vi "Read_Data_file.vi"(0 "Results file":path, 1 "Read Channel Names only":bool, 2 "Delete First Rows?":bool, 3 "Add Extra Channels?":bool, 5 "Template File":path, 7 "Run EnFlo Hub? (T)":bool=TRUE, 8 "Desired File Types":T1) -> (9 "Deleted Rows":string[][](array[string]), 10 "Row numbers":i32[](array[numeric]), 11 "Template File Out":path, 12 "Filetype":string, 14 "Results file Out":path, 15 "String Before":string, 16 "Ch names Out":string[](array[string]), 17 "Channel Values Out":string[][](array[string]), 18 "String After":string, 19 "Start Bytes":i32)   [LabVIEW 2022 SP3]
uses:
  Data_File_Type.ctl
  Globals/Meas_global.vi
panel:
  out "Case":string
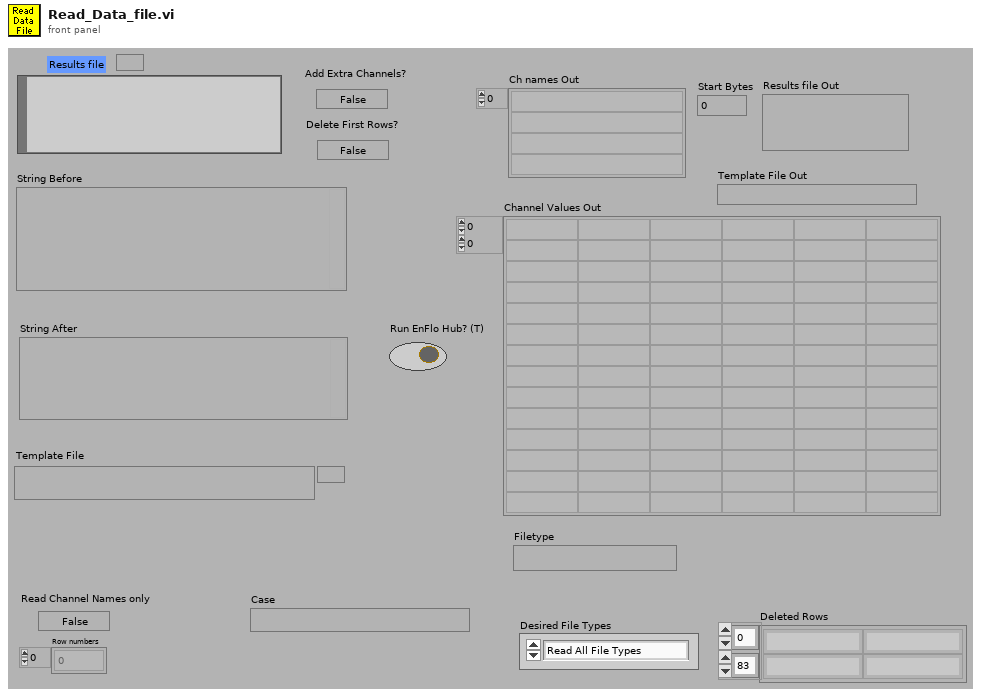
[diagram p1: front panel]
types:
  T1 = typedef "Data_File_Type.ctl" = enum16{"Read All File Types", "Results Files Only", "Raw Data Files Only", "Calibration Files Only", "Gas Desk Files Only", "Old Results Files Only", "Tabulated Data Files Only"}
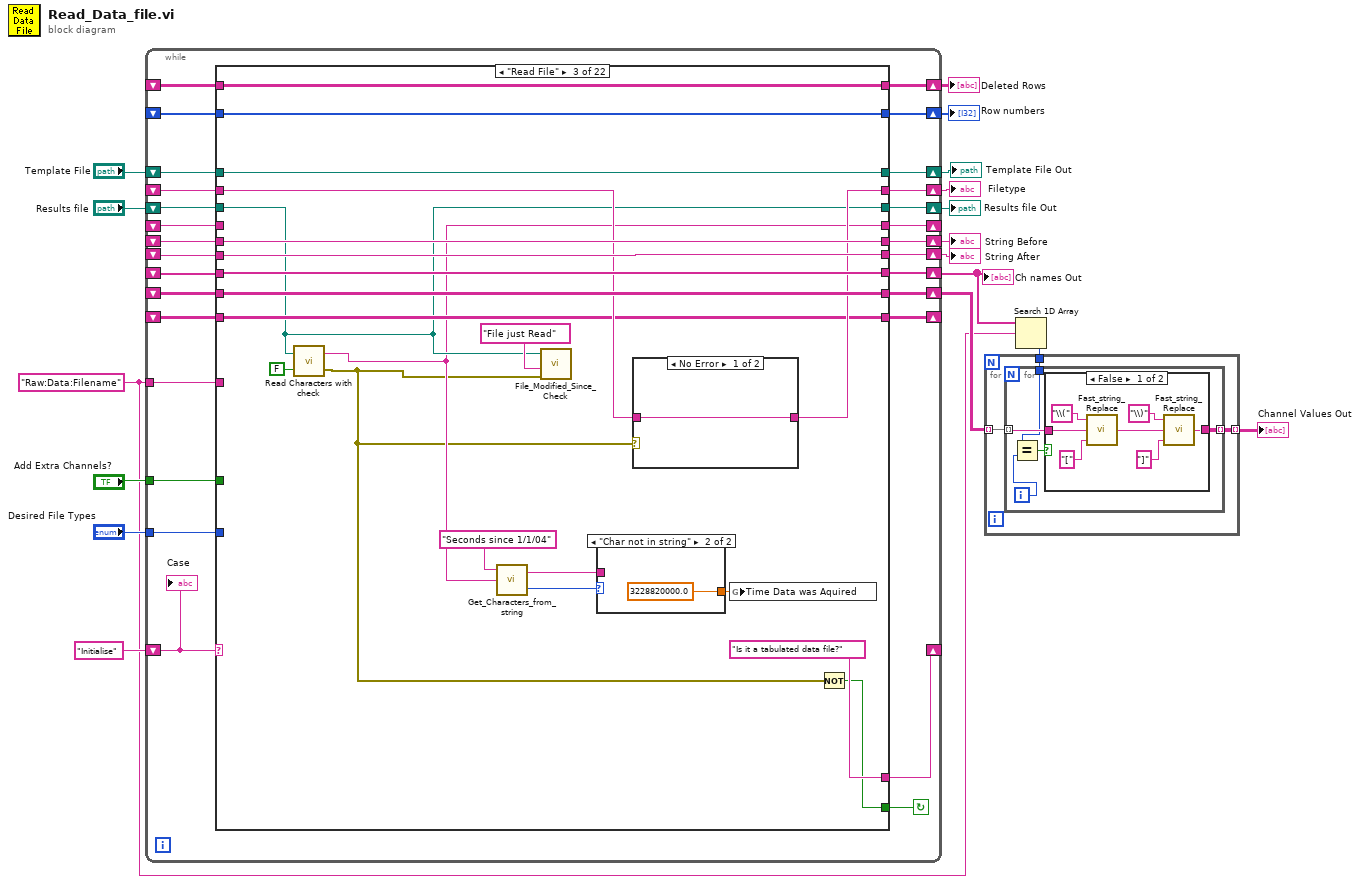
[diagram p0: block diagram]
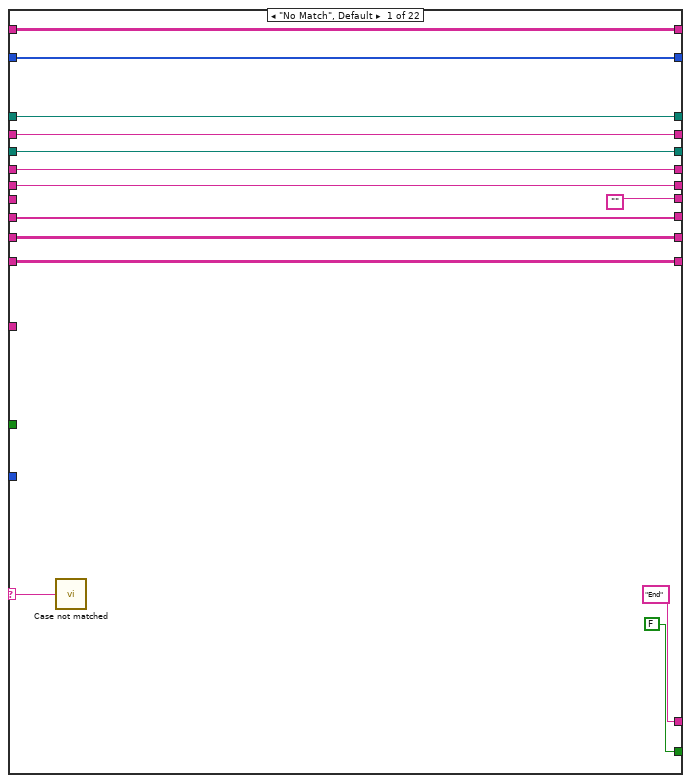
[diagram p3: hidden frame]
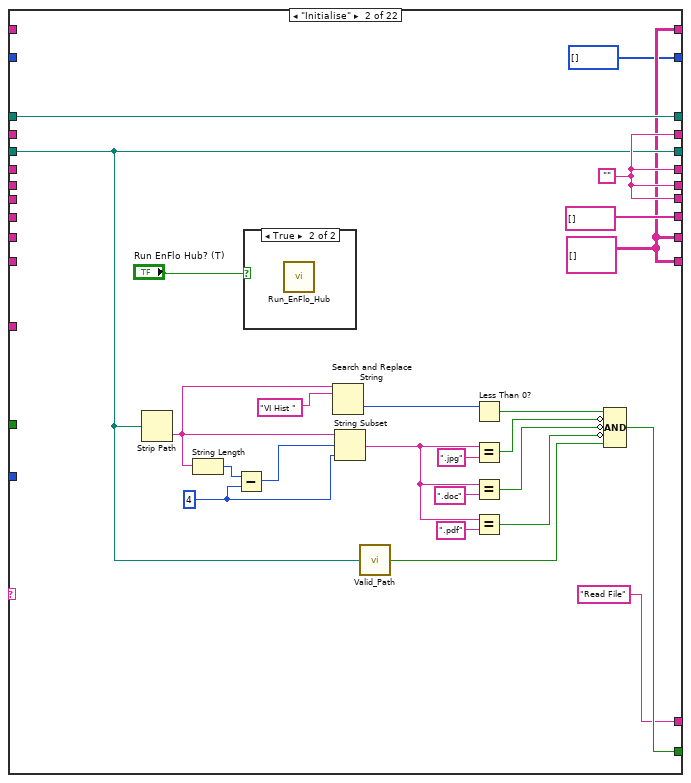
[diagram p4: hidden frame]
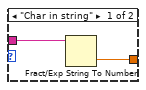
[diagram p6: hidden frame]
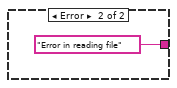
[diagram p7: hidden frame]
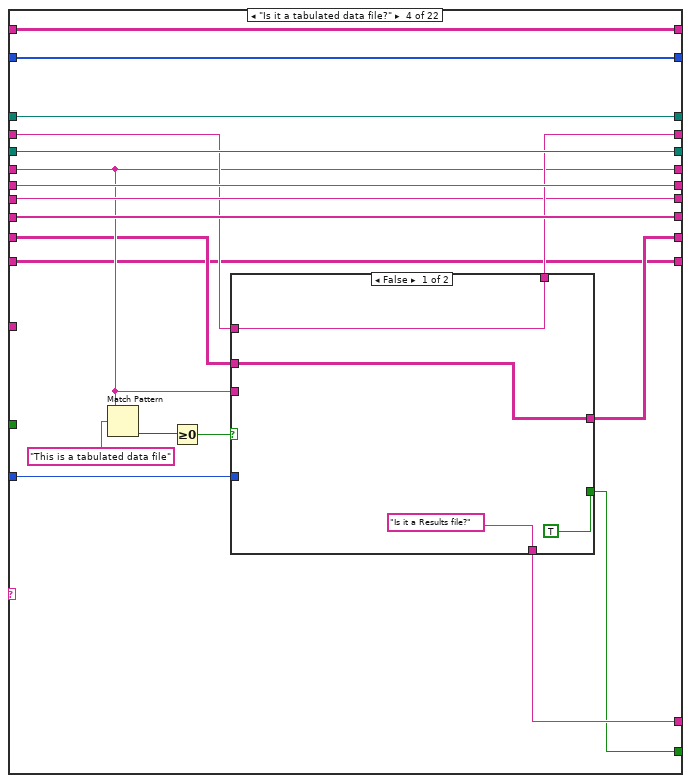
[diagram p8: hidden frame]
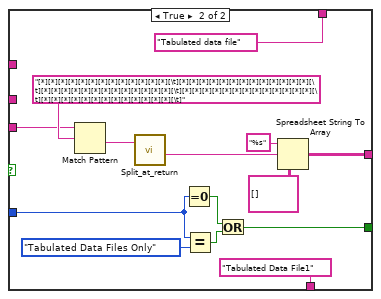
[diagram p9: hidden frame]
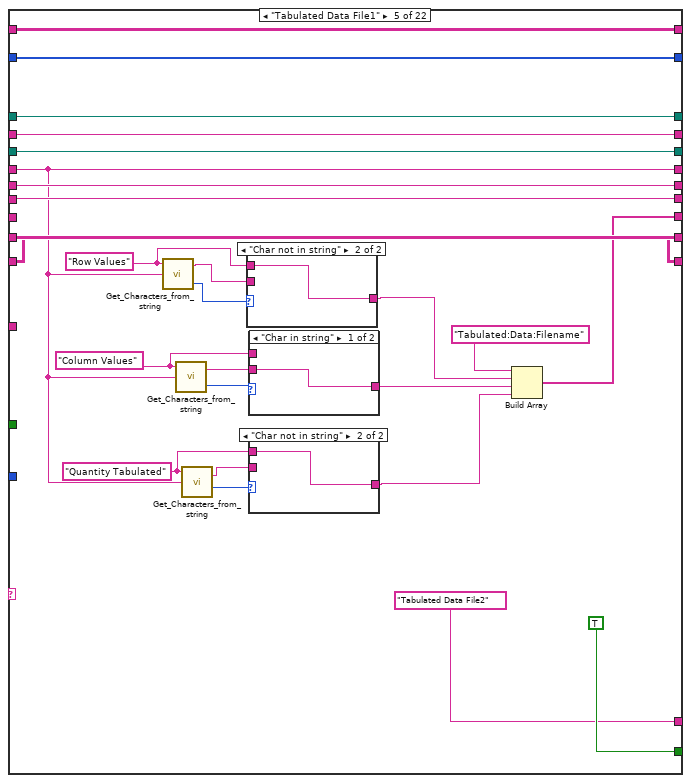
[diagram p10: hidden frame]
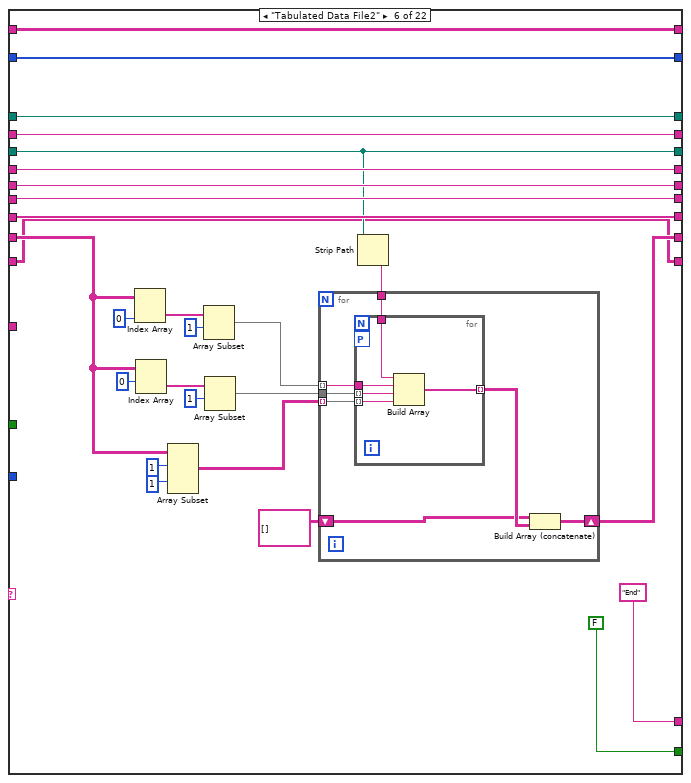
[diagram p14: hidden frame]
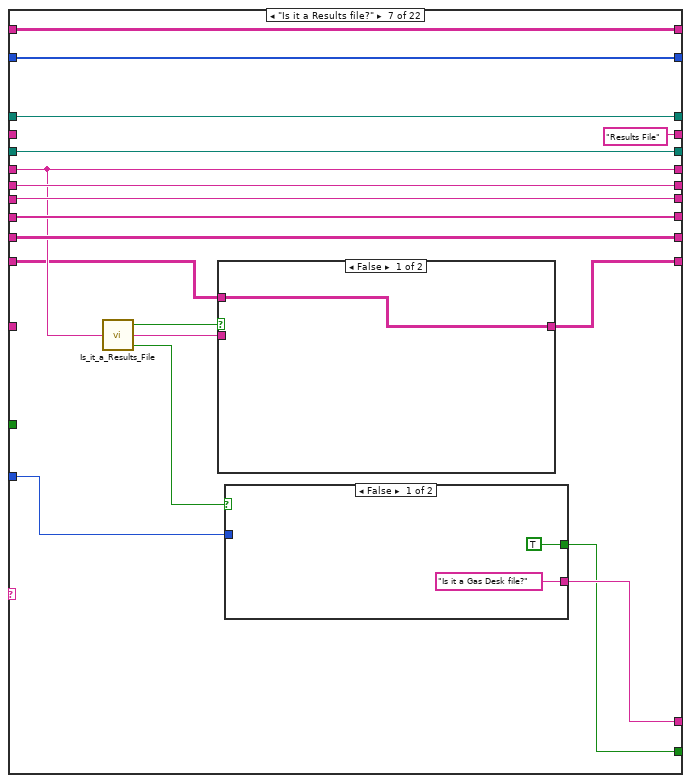
[diagram p15: hidden frame]
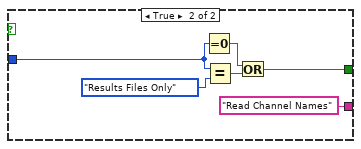
[diagram p16: hidden frame]
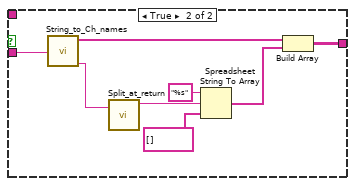
[diagram p17: hidden frame]
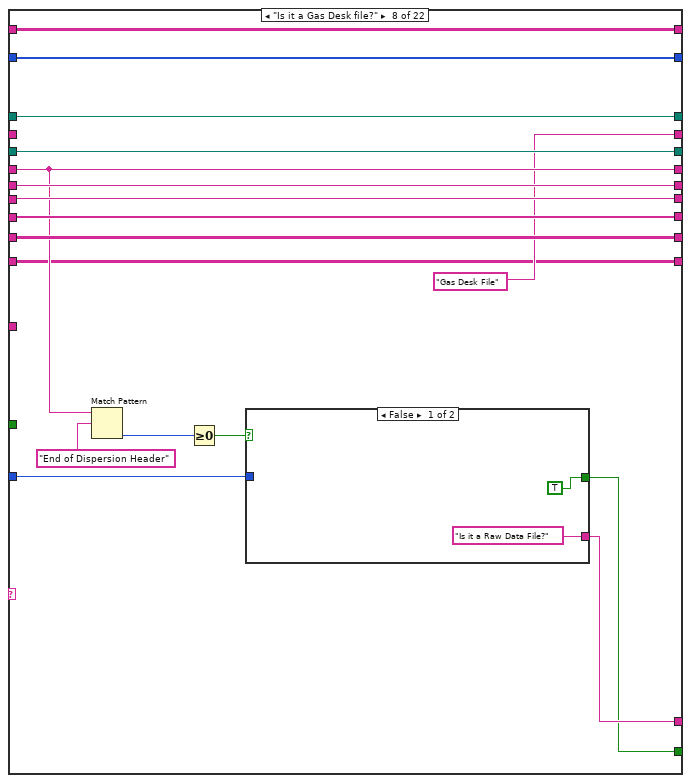
[diagram p18: hidden frame]
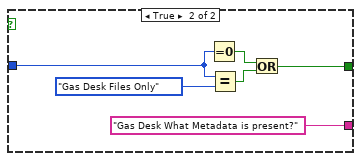
[diagram p19: hidden frame]
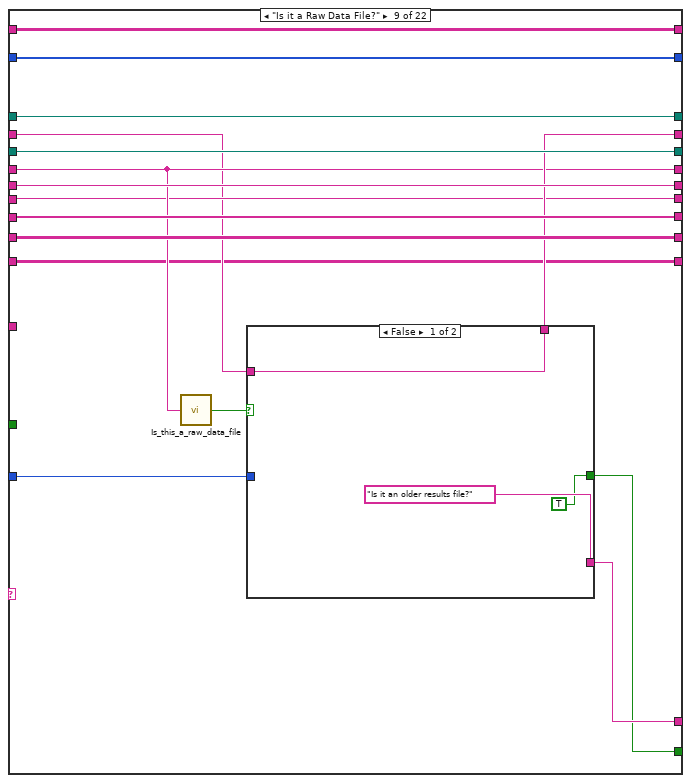
[diagram p20: hidden frame]
diagram:
  w2 = "Raw:Data:Filename"
  n1 = while {
    tunnel: "Add Extra Channels?" -> [w28]
    shift-left: _ -> [w32]
    shift-right: [w31] -> w16
    shift-left: "Results file" -> [w34]
    shift-right: [w33] -> w14
    shift-left: _ -> [w36]
    shift-right: [w35] -> w11
    shift-left: _ -> [w29]
    shift-right: [w37] -> w13
    shift-left: _ -> [w38]
    shift-right: [w39] -> _
    shift-left: "Initialise" -> [w42]
    shift-right: [w40] -> _
    shift-left: _ -> [w30]
    shift-right: [w44] -> w5
    shift-left: _ -> [w41]
    shift-right: [w45] -> w3
    shift-right: [w27] -> w10
    shift-left: "Template File" -> [w26]
    shift-right: [w24] -> w8
    shift-left: _ -> [w25]
    tunnel: "Desired File Types" -> [w23]
    shift-right: [w22] -> w6
    shift-left: _ -> [w21]
    shift-right: [w20] -> _
    shift-left: _ -> [w19]
    tunnel: w2 -> [w18]
    stop <- w43 continue-if-true
    n2 = case shown="\"Read File\"" w42 {
      selector: w42 -> [w47 _ _ _ _ _ _ _ _ _ _ _ _ _ _ _ _ _ _ _ _ _]
      tunnel: [w58 string[] [] ("Extra Channel Names") w103 w128 w154 w205 w235 w269 w293 w321 w355 w389 w410 w449 w477 w479 w560 w604 w654 w679 w702 w728] -> w45
      tunnel: [w57 w61 w102 w117 w172 w194 w234 w268 w292 w320 w354 w388 w409 w448 w476 w499 w566 w621 w653 w674 w696 w725] -> w44
      tunnel: [FALSE ("Results File?") w73 w99 w112 TRUE ("Results File?") FALSE ("Results File?") w226 w255 w281 w307 w341 w381 TRUE ("Results File?") TRUE ("Results File?") TRUE ("Results File?") w487 TRUE ("Results File?") TRUE ("Results File?") FALSE ("Results File?") TRUE ("Results File?") w697 FALSE ("Results File?")] -> w43
      tunnel: w41 -> [w58 _ w103 w128 _ w205 w235 w269 w293 w321 w355 w389 w410 w449 w477 _ w560 w605 w658 w679 w702 w730]
      tunnel: ["End" "Read File" "Is it a tabulated data file?" w124 "Tabulated Data File2" ("f") "End" ("f") w233 w256 w288 w316 "Read Channel Names" ("f") "Read Channel Names" ("f") w395 "Read Channel Names" ("f") "Read Channel Names" ("f") w490 "Does template file exist?" ("f") w616 "End" ("f") "Delete First Row?" ("f") "Add Extra Channels of data" ("f") "End" ("f")] -> w40
      tunnel: [w55 w82 w86 w118 w165 w201 w228 w262 w286 w311 w350 w377 w397 w428 w460 w492 w561 w620 w659 w672 w704 w732] -> w39
      tunnel: w38 -> [w55 _ _ w118 w165 w201 w228 w262 w286 w311 w350 w384 w396 w428 w460 w494 w561 w620 w659 w672 w704 w732]
      tunnel: [w54 w82 w101 w126 w170 w204 w229 w265 w290 w318 w353 w386 w406 w445 w474 w493 w558 w619 w662 w678 w707 w736] -> w37
      tunnel: w36 -> [_ _ w100 w123 w168 w202 w231 w266 w285 w315 w352 _ w407 w446 w475 w498 w565 w618 w661 w677 w706 w735]
      tunnel: ["" w82 w100 w123 w168 w202 w231 w266 w285 w315 w352 w374 w407 w446 w475 w498 w565 w618 w661 w677 w706 w735] -> w35
      tunnel: w34 -> [w53 w71 w87 w127 w171 w184 w232 w267 w291 w319 w335 w387 w408 w447 w456 w497 w564 w602 w657 w671 w703 w731]
      tunnel: [w53 w71 w87 w127 w171 w184 w232 w267 w291 w319 w335 w387 w408 w447 w456 w497 w564 w602 w657 w671 w703 w731] -> w33
      tunnel: w32 -> [w51 _ w97 w122 w167 w200 _ _ w284 w314 _ w380 w394 w443 w472 w496 w563 w617 w656 w668 w701 w734]
      tunnel: [w51 w82 w98 w125 w167 w200 "Results File" "Gas Desk File" w289 w317 w340 w380 w394 w443 w472 w496 w563 w617 w656 w668 w701 w734] -> w31
      tunnel: w30 -> [w57 _ w102 w116 w172 w193 w234 w268 w292 w320 w354 w388 w409 w448 w476 w499 w566 w621 _ _ w700 w727]
      tunnel: w29 -> [w54 _ w101 w126 w170 w204 w229 w265 w290 w318 w353 w386 w406 w445 w474 _ w558 w619 w662 w678 w707 w736]
      tunnel: w28 -> [_ _ _ _ _ _ _ _ _ _ w342 _ _ _ _ _ _ _ _ _ w692 _]
      tunnel: [w50 w72 w96 w115 w150 w182 w224 w260 w283 w309 w339 w371 w393 w426 w455 w488 w557 w599 w652 w667 w683 w724] -> w27
      tunnel: w26 -> [w50 w72 w96 w115 w150 w182 w224 w260 w283 w309 w339 w371 w393 w426 w455 w488 w557 w599 w651 w667 w683 w724]
      tunnel: [w49 i32[] [] ("Row numbers") w95 w114 w149 w181 w223 w259 w282 w308 w338 w370 w392 w425 w454 w483 w556 w612 w650 w666 w684 w723] -> w24
      tunnel: w25 -> [w49 _ w95 w114 w149 w181 w223 w259 w282 w308 w338 w370 w392 w425 w454 w483 w556 w612 _ w666 _ w723]
      tunnel: w23 -> [_ _ _ w113 _ _ w221 w258 w280 w306 w337 _ _ _ _ _ _ _ _ _ _ _]
      tunnel: [w48 w61 w90 w111 w148 w180 w220 w254 w279 w305 w333 w369 w391 w424 w453 w482 w555 w603 w649 w665 w691 w722] -> w22
      tunnel: w21 -> [w48 _ w90 w111 w148 w180 w220 w254 w279 w305 w333 w369 w391 w424 w453 w482 w555 w603 _ w665 w690 w722]
      tunnel: [w46 w61 w89 w110 w147 w179 w219 w253 w278 w304 w332 w368 w390 w421 w450 w481 w553 w595 w648 w664 w688 w718] -> w20
      tunnel: w19 -> [w46 _ w89 w110 w147 w179 w218 w253 w278 w304 w332 w368 w390 _ _ w481 w554 w591 w648 w664 w688 w718]
      tunnel: w18 -> [_ _ _ _ _ _ _ _ _ _ _ _ _ _ _ _ w552 _ _ _ _ _]
      frame "No Match", Default {
        n3 = call "Case not matched.vi"("Case Name not Matched"=w47) -> ()
      }
      frame "Initialise" {
        w80 = 4 ("length (rest)")
        w82 = ""
        w61 = string[][] [] ("Channel Values")
        n4 = Strip Path(path=w71) -> (name=w78:string)  [unwired: 1 out]
        n5 = String Length(string=w78) -> (length=w81:i32)
        n6 = Subtract(x=w81, y=w80) -> (x-y=w79:i32)
        n7 = case shown="True" "Run EnFlo Hub? (T)" {
          frame False {
          }
          frame True {
            n8 = call "Run_EnFlo_Hub.vi"() -> ()  [unwired: 1 in, 7 out]
          }
        }
        n9 = Search and Replace String(input string=w78, search string="VI Hist ") -> (offset past replacement=w76:i32)  [unwired: 1 in, 8 out]
        n10 = String Subset(string=w78, offset (0)=w79, length (rest)=w80) -> (substring=w66:string)
        n11 = call "Valid_Path.vi"("Filename"=w71) -> ("Valid Path?"=w63:bool)
        n12 = Less Than 0?(x=w76) -> (x < 0?=w74:bool)
        n13 = Equal?(x=w66, y=".jpg") -> (x = y?=w75:bool)
        n14 = Equal?(x=w66, y=".doc") -> (x = y?=w69:bool)
        n15 = Equal?(x=w66, y=".pdf") -> (x = y?=w65:bool)
        n16 = Compound Arithmetic op=AND(w74, invert w75, invert w69, invert w65, w63) -> (w73:bool)
      }
      frame "Read File" {
        n17 = call "Read Characters with check.vi"("Call EnFlo Error Handler?"=FALSE, "file (use dialog)"=w87) -> ("error out"=w85:errorcluster, "Read String"=w86:string)
        n18 = call "Get_Characters_from_string.vi"("Input string"=w86, "Variable name"="Seconds since 1/1/04") -> ("Status"=w91:enum16{"Char in string", "Char not in string"}, "Value"=w93:string)  [unwired: 1 in]
        n19 = call "File_Modified_Since_Check.vi"("error in"=w85, "mode"="File just Read", "File Path"=w87) -> ()  [unwired: 5 in, 2 out]
        n20 = case shown="\"Char not in string\"" w91 {
          tunnel: w93 -> [w106 _]
          tunnel: [w105 3228820000.0 ("y")] -> w92
          frame "Char in string" {
            n21 = Fract/Exp String To Number(string=w106) -> (number=w105:dbl)  [unwired: 4 out]
          }
          frame "Char not in string" {
          }
        }
        n22 = case shown="No Error" w85 {
          tunnel: [w108 "Error in reading file"] -> w98
          tunnel: w97 -> [w108 _]
          frame No Error {
          }
          frame Error {
          }
        }
        n23 = global write "Meas_global.vi" "Time Data was Aquired"(w92) -> ()
        n24 = Not(x=w85) -> (.not. x?=w99:bool)
      }
      frame "Is it a tabulated data file?" {
        n25 = Match Pattern(string=w118, regular expression="This is a tabulated data file") -> (offset past match=w121:i32)  [unwired: 4 out]
        n26 = Greater Or Equal To 0?(x=w121) -> (x >= 0?=w120:bool)
        n27 = case shown="False" w120 {
          tunnel: [w132 "Tabulated data file"] -> w125
          tunnel: ["Is it a Results file?" "Tabulated Data File1" ("f")] -> w124
          tunnel: w122 -> [w132 _]
          tunnel: w118 -> [_ w143]
          tunnel: [w131 w140] -> w117
          tunnel: w116 -> [w131 _]
          tunnel: w113 -> [_ w136]
          tunnel: [TRUE ("Results File?") w133] -> w112
          frame False {
          }
          frame True {
            n28 = Match Pattern(string=w143, regular expression="[*][*][*][*][*][*][*][*][*][*][*][*][*][\t][*][*][*][*][*][*][*][*][*][*][*][*][*][\t][*][*][*][*][*][*][*][*][*][*][*][*][*][\t][*][*][*][*][*][*][*][*][*][*][*][*][*][\t][*][*][*][*][*][*][*][*][*][*][*][*][*][\t]" ("String")) -> (after substring=w139:string)  [unwired: 4 out]
            n29 = call "Split_at_return.vi"("String"=w139) -> ("after substring"=w138:string)  [unwired: 1 in, 3 out]
            n30 = Equal To 0?(x=w136) -> (x = 0?=w134:bool)
            n31 = Equal?(x=w136, y=Data_File_Type."Tabulated Data Files Only" ("Desired File Types")) -> (x = y?=w135:bool)
            n32 = Or(x=w134, y=w135) -> (x .or. y?=w133:bool)
            n33 = Spreadsheet String To Array(format string="%s", spreadsheet string=w138, array type (2D Dbl)=string[][] [] ("Channel Values")) -> (array=w140:string[][])  [unwired: 1 out]
          }
        }
      }
      frame "Tabulated Data File1" {
        w153 = "Row Values" ("Variable name")
        w152 = "Column Values" ("Variable name")
        w159 = "Quantity Tabulated" ("Variable name")
        n34 = call "Get_Characters_from_string.vi"("Input string"=w165, "Variable name"=w153) -> ("Status"=w157:enum16{"Char in string", "Char not in string"}, "Value"=w158:string)  [unwired: 1 in]
        n35 = call "Get_Characters_from_string.vi"("Input string"=w165, "Variable name"=w152) -> ("Status"=w164:enum16{"Char in string", "Char not in string"}, "Value"=w163:string)  [unwired: 1 in]
        n36 = call "Get_Characters_from_string.vi"("Input string"=w165, "Variable name"=w159) -> ("Status"=w161:enum16{"Char in string", "Char not in string"}, "Value"=w160:string)  [unwired: 1 in]
        n37 = case shown="\"Char not in string\"" w157 {
          tunnel: w158 -> [w175 _]
          tunnel: [w175 w176] -> w156
          tunnel: w153 -> [_ w176]
          frame "Char in string" {
          }
          frame "Char not in string" {
          }
        }
        n38 = case shown="\"Char in string\"" w164 {
          tunnel: w163 -> [w177 _]
          tunnel: [w177 w178] -> w162
          tunnel: w152 -> [_ w178]
          frame "Char in string" {
          }
          frame "Char not in string" {
          }
        }
        n39 = case shown="\"Char not in string\"" w161 {
          tunnel: w160 -> [w173 _]
          tunnel: [w173 w174] -> w155
          tunnel: w159 -> [_ w174]
          frame "Char in string" {
          }
          frame "Char not in string" {
          }
        }
        n40 = Build Array("Tabulated:Data:Filename", w156, w162, w155) -> (w154:string[])
      }
      frame "Tabulated Data File2" {
        n41 = Index Array(array=w193, index (col)=0 ("index (row)")) -> (element=w188:string[])  [unwired: 1 in]
        n42 = Index Array(array=w193, index (row)=0) -> (element=w192:string[])  [unwired: 1 in]
        n43 = Array Subset(array=w193, index (row)=1 ("index"), index (col)=1 ("index")) -> (w196:string[][])  [unwired: 2 in]
        n44 = Array Subset(array=w188, index=1) -> (w187:string[])  [unwired: 1 in]
        n45 = Array Subset(array=w192, index=1) -> (w189:string[])  [unwired: 1 in]
        n46 = Strip Path(path=w184) -> (name=w183:string)  [unwired: 1 out]
        n47 = for {
          tunnel: w187 -> [w212] mode=indexing
          tunnel: w189 -> [w211]
          tunnel: w196 -> [w210] mode=indexing
          shift-right: [w207] -> w194
          shift-left: string[][] [] -> [w208]
          tunnel: w183 -> [w206]
          n48 = for {
            tunnel: w212 -> [w217]
            tunnel: w211 -> [w216] mode=indexing
            tunnel: w210 -> [w215] mode=indexing
            tunnel: [w214] -> w209 mode=indexing
            tunnel: w206 -> [w213]
            workers-P: _ -> [_]
            n49 = Build Array(w213, w217, w216, w215) -> (w214:string[])
          }
          n50 = Build Array (concatenate)(w208, w209) -> (w207:string[][])
        }
      }
      frame "Is it a Results file?" {
        n51 = call "Is_it_a_Results_File.vi"("character string"=w228) -> ("Contain DB Header Info"=w227:bool, "Header String"=w222:string, "Results File?"=w225:bool)
        n52 = case shown="False" w227 {
          tunnel: w222 -> [_ w248]
          tunnel: [w244 w245] -> w219
          tunnel: w218 -> [w244 _]
          frame False {
          }
          frame True {
            n53 = call "String_to_Ch_names.vi"("Spreadsheet string"=w248) -> ("Ch names"=w247:string[], "String After names"=w251:string)  [unwired: 2 out]
            n54 = call "Split_at_return.vi"("String"=w251) -> ("before substring"=w252:string)  [unwired: 1 in, 3 out]
            n55 = Spreadsheet String To Array(format string="%s", spreadsheet string=w252, array type (2D Dbl)=string[] [] ("Channel Values")) -> (array=w246:string[])  [unwired: 1 out]
            n56 = Build Array(w247, w246) -> (w245:string[][])
          }
        }
        n57 = case shown="False" w225 {
          tunnel: ["Is it a Gas Desk file?" "Read Channel Names"] -> w233
          tunnel: w221 -> [_ w240]
          tunnel: [TRUE w238] -> w226
          frame False {
          }
          frame True {
            n58 = Equal To 0?(x=w240) -> (x = 0?=w241:bool)
            n59 = Equal?(x=w240, y=Data_File_Type."Results Files Only" ("Desired File Types")) -> (x = y?=w242:bool)
            n60 = Or(x=w241, y=w242) -> (x .or. y?=w238:bool)
          }
        }
      }
      frame "Is it a Gas Desk file?" {
        n61 = Match Pattern(string=w262, regular expression="End of Dispersion Header") -> (offset past match=w264:i32)  [unwired: 4 out]
        n62 = Greater Or Equal To 0?(x=w264) -> (x >= 0?=w257:bool)
        n63 = case shown="False" w257 {
          tunnel: ["Is it a Raw Data File?" "Gas Desk What Metadata is present?"] -> w256
          tunnel: w258 -> [_ w274]
          tunnel: [TRUE w272] -> w255
          frame False {
          }
          frame True {
            n64 = Equal To 0?(x=w274) -> (x = 0?=w275:bool)
            n65 = Equal?(x=w274, y=Data_File_Type."Gas Desk Files Only" ("Desired File Types")) -> (x = y?=w276:bool)
            n66 = Or(x=w275, y=w276) -> (x .or. y?=w272:bool)
          }
        }
      }
      frame "Is it a Raw Data File?" {
        n67 = call "Is_this_a_raw_data_file.vi"("character string"=w286) -> ("Raw Dat File?"=w287:bool)  [unwired: 2 out]
        n68 = case shown="False" w287 {
          tunnel: [w295 "Raw Data File"] -> w289
          tunnel: ["Is it an older results file?" ("f") "Does Raw data file Contain ADAM data?" ("f")] -> w288
          tunnel: w284 -> [w295 _]
          tunnel: [TRUE ("Results File?") w298] -> w281
          tunnel: w280 -> [_ w299]
          frame False {
          }
          frame True {
            n69 = Equal To 0?(x=w299) -> (x = 0?=w301:bool)
            n70 = Equal?(x=w299, y=Data_File_Type."Raw Data Files Only" ("Desired File Types")) -> (x = y?=w300:bool)
            n71 = Or(x=w301, y=w300) -> (x .or. y?=w298:bool)
          }
        }
      }
      frame "Is it an older results file?" {
        n72 = Match Pattern(string=w311, regular expression="Date of meas\tTime of meas") -> (offset past match=w312:i32)  [unwired: 4 out]
        n73 = Greater Or Equal To 0?(x=w312) -> (x >= 0?=w310:bool)
        n74 = case shown="False" w310 {
          tunnel: [w324 "Older Results File"] -> w317
          tunnel: ["Is it a calibration file?" ("f") "Read Channel Names" ("f")] -> w316
          tunnel: w314 -> [w324 _]
          tunnel: [TRUE ("Results File?") w326] -> w307
          tunnel: w306 -> [_ w325]
          frame False {
          }
          frame True {
            n75 = Equal To 0?(x=w325) -> (x = 0?=w329:bool)
            n76 = Equal?(x=w325, y=Data_File_Type."Old Results Files Only" ("Desired File Types")) -> (x = y?=w328:bool)
            n77 = Or(x=w329, y=w328) -> (x .or. y?=w326:bool)
          }
        }
      }
      frame "Is it a calibration file?" {
        w349 = FALSE  # Show Dialog?
        n78 = Format Into String(format string="Data File   %s", w335) -> (resulting string=w334:string)  [unwired: 2 in, 1 out]
        n79 = call "2D_array_from_string.vi"("String Name"=w334, "Show Dialog?"=w349, "Input string"=w350, "Array title"="Calib points label") -> ("2D data array"=w348:dbl[][])
        n80 = Array Size(array=w348) -> (size(s)=w347:i32[])
        n81 = Index Array(array=w347, index=0 ("Index")) -> (element=w345:i32)
        n82 = Greater Than 0?(x=w345) -> (x > 0?=w343:bool)
        n83 = case shown="False" w343 {
          tunnel: w342 -> [_ w367]
          tunnel: [w356 w359] -> w341
          tunnel: ["File with no header" "Calibration File"] -> w340
          tunnel: w337 -> [w357 w363]
          frame False {
            n84 = Equal To 0?(x=w357) -> (x = 0?=w356:bool)
          }
          frame True {
            n85 = Not(x=w367) -> (.not. x?=w360:bool)
            n86 = Equal To 0?(x=w363) -> (x = 0?=w365:bool)
            n87 = Equal?(x=w363, y=Data_File_Type."Calibration Files Only" ("Desired File Types")) -> (x = y?=w364:bool)
            n88 = Or(x=w365, y=w364) -> (x .or. y?=w361:bool)
            n89 = Or(x=w360, y=w361) -> (x .or. y?=w359:bool)
          }
        }
      }
      frame "Does Raw data file Contain ADAM data?" {
        w372 = "\r\n"
        w375 = "Raw data header Start"
        n90 = Match Pattern(string=w384, regular expression=w375) -> (before substring=w378:string, after substring=w373:string)  [unwired: 3 out]
        n91 = Match Pattern(string=w378, regular expression="[*][*][*][*][*][*][*][*][*][*][*][*][*][*][*][*][*][*][*][*][*]" ("String")) -> (before substring=w377:string)  [unwired: 4 out]
        n92 = Concatenate Strings(w372, "************************", w372, w375, w373) -> (w374:string)
        n93 = String Length(string=w378) -> (length=w383:i32)
        n94 = Greater?(x=w383, y=30) -> (0:w381:bool)
      }
      frame "Gas Desk What Metadata is present?" {
        n95 = String Subset(string=w396, offset (0)=0, length (rest)=6 ("length")) -> (substring=w403:string)
        n96 = Equal?(x="******", y=w403) -> (x = y?=w401:bool)
        n97 = case shown="False" w401 {
          tunnel: [w412 "Gas Desk Read ADAM ch's Header"] -> w395
          tunnel: w396 -> [w411 _]
          frame False {
            w416 = "Data Base\tData Base\tData Base\t"
            n98 = String Length(string=w416) -> (length=w419:i32)
            n99 = String Subset(string=w411, offset (0)=0, length (rest)=w419) -> (substring=w417:string)
            n100 = Equal?(x=w416, y=w417) -> (x = y?=w415:bool)
            n101 = Select(t="Gas Desk DB Header Present", s=w415, f="Read Channel Names") -> (s? t:f=w412:string)
          }
          frame True {
          }
        }
        n102 = call "Fast_string_Replace.vi"("Replace match with:"="Suspect Pulse Width" ("regular expression"), "Input String"=w396, "regular expression"="Suspect \u0003Pulse Width ") -> ("Output String"=w397:string)  [unwired: 2 out]
      }
      frame "Gas Desk DB Header Present" {
        w430 = string[] [] ("Channel Values")
        n103 = call "String_to_Ch_names.vi"("Spreadsheet string"=w428) -> ("Ch names"=w442:string[], "String After names"=w431:string)  [unwired: 2 out]
        n104 = call "Split_at_return.vi"("String"=w431) -> ("before substring"=w433:string, "after substring"=w434:string)  [unwired: 1 in, 2 out]
        n105 = call "Split_at_return.vi"("String"=w434) -> ("after substring"=w435:string)  [unwired: 1 in, 3 out]
        n106 = call "String_to_Ch_names.vi"("Spreadsheet string"=w435) -> ("Ch names"=w441:string[], "String After names"=w436:string)  [unwired: 2 out]
        n107 = call "Split_at_return.vi"("String"=w436) -> ("after substring"=w438:string)  [unwired: 1 in, 3 out]
        n108 = call "Split_at_return.vi"("String"=w438) -> ("before substring"=w439:string)  [unwired: 1 in, 3 out]
        n109 = Spreadsheet String To Array(format string="%s", spreadsheet string=w439, array type (2D Dbl)=w430) -> (array=w440:string[])  [unwired: 1 out]
        n110 = Build Array (concatenate)(w441, w442) -> (w423:string[])
        n111 = Spreadsheet String To Array(format string="%s", spreadsheet string=w433, array type (2D Dbl)=w430) -> (array=w429:string[])  [unwired: 1 out]
        n112 = Build Array (concatenate)(w440, w429) -> (w422:string[])
        n113 = Build Array(w423, w422) -> (w421:string[][])
      }
      frame "Gas Desk Read ADAM ch's Header" {
        n114 = call "Split_at_return.vi"("String"=w460) -> ("after substring"=w468:string)  [unwired: 1 in, 3 out]
        n115 = call "String_to_Ch_names.vi"("Spreadsheet string"=w468) -> ("Ch names"=w457:string[], "String After names"=w469:string)  [unwired: 2 out]
        n116 = call "Split_at_return.vi"("String"=w469) -> ("after substring"=w470:string)  [unwired: 1 in, 3 out]
        n117 = call "Split_at_return.vi"("String"=w470) -> ("before substring"=w467:string)  [unwired: 1 in, 3 out]
        n118 = Spreadsheet String To Array(format string="%s", spreadsheet string=w467, array type (2D Dbl)=string[] [] ("Channel Values")) -> (array=w461:string[])  [unwired: 1 out]
        n119 = Strip Path(path=w456) -> (stripped path=w463:path, name=w462:string)
        n120 = Path To String(path=w463) -> (string=w464:string)
        n121 = Build Array (concatenate)("Original:Results:Filename", "Original:Results:Filepath", w457) -> (w452:string[])
        n122 = Build Array (concatenate)(w462, w464, w461) -> (w451:string[])
        n123 = Build Array(w452, w451) -> (w450:string[][])
      }
      frame "Read Channel Names" {
        n124 = case shown="\"File with no header\", Default" w496 {
          tunnel: [w513 w527 w536 0 0] -> w484
          tunnel: [w512 w526 w540 w545 w550] -> w491
          tunnel: w494 -> [w511 w528 w539 w548 w550]
          tunnel: [w510 w534 "Is Raw Data Filename Present?" ("f") w543 w549] -> w490
          tunnel: "Does template file exist?" ("f") -> [w510 w534 _ w543 w549]
          frame "Results File" {
            n125 = Match Pattern(string=w511, regular expression="[*][*][*][*][*][*][*][*][*][*][*][*][*][\t][*][*][*][*][*][*][*][*][*][*][*][*][*][\t][*][*][*][*][*][*][*][*][*][*][*][*][*][\t][*][*][*][*][*][*][*][*][*][*][*][*][*][\t][*][*][*][*][*][*][*][*][*][*][*][*][*][\t]" ("String")) -> (after substring=w516:string, offset past match=w514:i32)  [unwired: 3 out]
            n126 = call "Split_at_return.vi"("String"=w516) -> ("after substring"=w512:string, "offset past match"=w515:i32)  [unwired: 1 in, 2 out]
            n127 = Add(x=w514, y=w515) -> (x+y=w513:i32)
          }
          frame "Older Results File" {
            w521 = "\r"
            n128 = Match Pattern(string=w528, regular expression="Date of meas\tTime of meas") -> (before substring=w532:string, match substring=w525:string, offset past match=w529:i32)  [unwired: 2 out]
            n129 = Reverse String(1:w532) -> (0:w531:string)
            n130 = String Length(string=w525) -> (length=w524:i32)
            n131 = Match Pattern(string=w531, regular expression=w521) -> (after substring=w530:string, offset past match=w522:i32)  [unwired: 3 out]
            n132 = Match Pattern(string=w530, regular expression=w521) -> (after substring=w520:string, offset past match=w523:i32)  [unwired: 3 out]
            n133 = Match Pattern(string=w520, regular expression=w521) -> (offset past match=w519:i32)  [unwired: 4 out]
            n134 = Compound Arithmetic op=ADD(invert w524, w529, invert w523, invert w522, invert w519, 1 ("value")) -> (w527:i32)
            n135 = Search/Split String(string=w528, offset (0)=w527) -> (match + rest of string=w526:string)  [unwired: 3 out]
          }
          frame "Gas Desk File" {
            n136 = Match Pattern(string=w539, regular expression="End of Dispersion Header") -> (after substring=w542:string, offset past match=w537:i32)  [unwired: 3 out]
            n137 = call "Split_at_return.vi"("String"=w542) -> ("after substring"=w540:string, "offset past match"=w538:i32)  [unwired: 1 in, 2 out]
            n138 = Add(x=w538, y=w537) -> (x+y=w536:i32)
          }
          frame "Raw Data File" {
            n139 = Search/Split String(string=w548, offset (0)=37 ("y")) -> (match + rest of string=w547:string)  [unwired: 3 out]
            n140 = call "Split_at_return.vi"("String"=w547) -> ("after substring"=w545:string)  [unwired: 1 in, 3 out]
          }
          frame "File with no header", Default {
          }
        }
        n141 = call "String_to_Ch_names.vi"("Spreadsheet string"=w491) -> ("Ch names"=w480:string[], "Title length (Bytes)"=w485:i32, "String After names"=w492:string)  [unwired: 1 out]
        n142 = case shown="False" "Read Channel Names only" {
          tunnel: w485 -> [_ w504]
          tunnel: w484 -> [_ w503]
          tunnel: w481 -> [_ w508]
          tunnel: w480 -> [w501 w507]
          tunnel: [w501 w505] -> w479
          tunnel: [0 w502] -> w478
          frame False {
          }
          frame True {
            n143 = Index Array(array=w508, index (row)=0) -> (element=w506:string[])  [unwired: 1 in]
            n144 = Add(x=w503, y=w504) -> (x+y=w502:i32)
            n145 = Build Array (concatenate)(w507, w506) -> (w505:string[])
          }
        }
        "Start Bytes" <- w478
        n146 = String Subset(string=w494, offset (0)=0, length (rest)=w484) -> (substring=w493:string)
        n147 = Not(x="Read Channel Names only") -> (.not. x?=w487:bool)
      }
      frame "Is Raw Data Filename Present?" {
        n148 = Search 1D Array(1D array=w560, element=w552) -> (index of element=w559:i32)  [unwired: 1 out]
        n149 = case shown="-1" w559 {
          tunnel: w558 -> [_ w580]
          tunnel: w552 -> [_ w573]
          tunnel: w554 -> [w568 w571]
          tunnel: [w568 w569] -> w553
          frame 0, Default {
          }
          frame -1 {
            n150 = Concatenate Strings("Raw data Directory", "\t") -> (w577:string)
            n151 = Match Pattern(string=w580, regular expression=w577) -> (after substring=w576:string)  [unwired: 4 out]
            n152 = call "Split_at_return.vi"("String"=w576) -> ("before substring"=w574:string)  [unwired: 1 in, 3 out]
            n153 = Match Pattern(string=w574, regular expression="\t") -> (before substring=w572:string)  [unwired: 4 out]
            n154 = Build Array(w573, w572) -> (w570:string[])
            n155 = for {
              tunnel: w571 -> [w583] mode=indexing
              tunnel: w570 -> [w582] mode=indexing
              tunnel: [w581] -> w569 mode=indexing
              workers-P: _ -> [_]
              n156 = Build Array (concatenate)(w583, w582) -> (w581:string[])
            }
          }
        }
      }
      frame "Does template file exist?" {
        n157 = Index Array(array=w591, index (row)=1) -> (element=w588:string[])  [unwired: 1 in]
        n158 = call "Common_Extra_Chs.vi"() -> ("Common Extra Channels"=w594:string[])
        n159 = while {
          shift-right: [w646] -> w610
          shift-left: _ -> [w647]
          stop <- TRUE stop-if-true
          n160 = Increment(x=w647) -> (x+1=w646:dbl)
        }
        n161 = Index Array(array=w591, index (row)=0) -> (element=w593:string[])  [unwired: 1 in]
        n162 = call "Does_file_exist_(simple).vi"("Pathname"=w599) -> ("exists?"=w600:bool)
        n163 = Path to Array of Strings(0:w602) -> (2:w615:string[])  [unwired: 1 out]
        n164 = case shown="True" w600 {
          tunnel: w599 -> [_ w644]
          tunnel: ["No Template File" w638] -> w598
          frame False {
          }
          frame True {
            n165 = File/Directory Info(path=w644) -> (last mod=w643:timestamp)  [unwired: 1 in, 6 out]
            n166 = Strip Path(path=w644) -> (name=w639:string)  [unwired: 1 out]
            n167 = Get Date/Time String(seconds (now)=w643) -> (date string=w640:string, time string=w641:string)  [unwired: 2 in]
            n168 = Format Into String(format string="%s last mod %s %s", w639, w640, w641) -> (resulting string=w638:string)  [unwired: 2 in, 1 out]
          }
        }
        n169 = Path To String(path=w602) -> (string=w601:string)
        n170 = Reverse 1D Array(array=w615) -> (reversed array=w614:string[])
        n171 = Array Subset(array=w614, length=5) -> (w613:string[])  [unwired: 1 in]
        n172 = Number To Decimal String(number=w610) -> (decimal integer string=w609:string)  [unwired: 1 out]
        n173 = Build Array (concatenate)(w613, w609, w601, w598) -> (w589:string[])
        n174 = for {
          tunnel: w593 -> [w629]
          tunnel: w594 -> [w627] mode=indexing
          tunnel: [w627] -> w592 mode=indexing if=w623
          shift-right: [w625] -> w587
          shift-left: w588 -> [w626]
          tunnel: w589 -> [w624] mode=indexing
          tunnel: [w624] -> w586 mode=indexing if=w623
          n175 = Search 1D Array(1D array=w629, element=w627) -> (index of element=w628:i32)  [unwired: 1 in]
          n176 = case shown="Default" w628 {
            selector: w628 -> [w633 _]
            tunnel: w626 -> [w634 w635]
            tunnel: w624 -> [w632 _]
            tunnel: [w631 w635] -> w625
            tunnel: [FALSE TRUE] -> w623
            frame Default {
              n177 = Replace Array Subset(array=w634, new element=w632, index=w633) -> (w631:string[])
            }
            frame -1 {
            }
          }
        }
        n178 = Build Array (concatenate)(w593, w592) -> (w585:string[])
        n179 = Build Array (concatenate)(w587, w586) -> (w584:string[])
        n180 = call "Update_Ch_Names.vi"("Ch Name in"=w605) -> ("Ch Name Out"=w604:string[])
        n181 = call "Valid_Path.vi"("Filename"=w599) -> ("Valid Path?"=w606:bool)
        n182 = call "Update_Ch_Names.vi"("Ch Name in"=w585) -> ("Ch Name Out"=w590:string[])
        n183 = Select(t="Read Values using Template", s=w606, f="Entire string to 2D array") -> (s? t:f=w616:string)
        n184 = Build Array(w590, w584) -> (w595:string[][])
      }
      frame "Read Values using Template" {
        n185 = call "Filter_on_template_file_new.vi"("Template File"=w651, "Extra Channel Values"=w648, "Filetype"=w656, "Channel Names In"=w658, "Data string"=w659, "Filename"=w657) -> ("Template File-write"=w652:path, "Row numbers"=w650:i32[], "Channel Names Out"=w654:string[], "Deleted Rows"=w649:string[][], "Data Out"=w655:string[][])  [unwired: 5 in]
        n186 = call "Surface_modularity.vi"("Data in"=w655, "Channel names"=w654) -> ("Data out"=w653:string[][])  [unwired: 1 out]
      }
      frame "Entire string to 2D array" {
        n187 = case shown="\"False\", Default" w668 {
          tunnel: [w680 w681] -> w673
          tunnel: w672 -> [w680 w681]
          frame "False", Default {
          }
          frame "Raw Data File" {
          }
        }
        n188 = Spreadsheet String To Array(format string="%s", spreadsheet string=w673, array type (2D Dbl)=string[][] [] ("Channel Values")) -> (array=w674:string[][])  [unwired: 1 out]
      }
      frame "Delete First Row?" {
        n189 = Index Array(array=w688, index (row)=0) -> (element=w687:string[])  [unwired: 1 in]
        n190 = Array Size(array=w687) -> (size(s)=w699:i32)
        n191 = Greater Than 0?(x=w699) -> (x > 0?=w698:bool)
        n192 = case shown="True" "Delete First Rows?" {
          tunnel: w701 -> [_ w712]
          tunnel: w700 -> [w710 w715]
          tunnel: [w710 w714] -> w696
          tunnel: [w709 w713] -> w691
          tunnel: w690 -> [w709 _]
          tunnel: [0 ("Rows removed") w711] -> w686
          frame False {
          }
          frame True {
            n193 = call "Delete_First_Rows.vi"("File Type"=w712, "Data In"=w715) -> ("Rows removed"=w711:i32, "Deleted Rows"=w713:string[][], "Data Out"=w714:string[][])
          }
        }
        n194 = And(x=w698, y=w692) -> (x .and. y?=w697:bool)
        n195 = Array Size(array=w696) -> (size(s)=w695:i32[])
        n196 = Index Array(array=w695, index=0) -> (element=w693:i32)
        n197 = for {
          N: w693 -> [_]
          tunnel: [w716] -> w685 mode=indexing
          workers-P: _ -> [_]
          i -> [w716]
        }
        n198 = Add(x=w686, y=w685) -> (x+y=w684:i32[])
      }
      frame "Add Extra Channels of data" {
        n199 = Index Array(array=w718, index (row)=0) -> (element=w719:string[])  [unwired: 1 in]
        n200 = Index Array(array=w718, index (row)=1) -> (element=w717:string[])  [unwired: 1 in]
        n201 = for {
          tunnel: w719 -> [w746] mode=indexing
          shift-right: [w744] -> w726
          shift-left: string[] [] -> [w745]
          shift-right: [w747] -> w728
          shift-left: w730 -> [w742]
          tunnel: w717 -> [w743] mode=indexing
          n202 = Search 1D Array(1D array=w742, element=w746) -> (index of element=w741:i32)  [unwired: 1 out]
          n203 = case shown="0, Default" w741 {
            selector: w741 -> [w748 _]
            tunnel: w742 -> [w752 w758]
            tunnel: [w752 w757] -> w747
            tunnel: w746 -> [_ w756]
            tunnel: w745 -> [w751 w755]
            tunnel: [w750 w754] -> w744
            tunnel: w743 -> [w749 w753]
            frame 0, Default {
              n204 = Replace Array Subset(array=w751, new element=w749, index=w748) -> (w750:string[])
            }
            frame -1 {
              n205 = Build Array (concatenate)(w758, w756) -> (w757:string[])
              n206 = Build Array (concatenate)(w755, w753) -> (w754:string[])
            }
          }
        }
        n207 = for {
          tunnel: w727 -> [w738] mode=indexing
          tunnel: w726 -> [w740]
          tunnel: [w739] -> w725 mode=indexing
          workers-P: _ -> [_]
          n208 = Build Array (concatenate)(w738, w740) -> (w739:string[])
        }
      }
    }
    "Case" <- w42
  }
  "Filetype" <- w16
  "Results file Out" <- w14
  "Ch names Out" <- w3
  "String Before" <- w13
  "String After" <- w11
  "Template File Out" <- w10
  "Row numbers" <- w8
  "Deleted Rows" <- w6
  n209 = Search 1D Array(1D array=w3, element=w2) -> (index of element=w1:i32)  [unwired: 1 out]
  n210 = for {
    tunnel: w5 -> [w761] mode=indexing
    tunnel: [w760] -> w4 mode=indexing
    tunnel: w1 -> [w759]
    n211 = for {
      tunnel: w761 -> [w766] mode=indexing
      tunnel: [w765] -> w760 mode=indexing
      tunnel: w759 -> [w763]
      i -> [w762]
      n212 = Equal?(x=w763, y=w762) -> (x = y?=w764:bool)
      n213 = case shown="False" w764 {
        tunnel: w766 -> [w768 w774]
        tunnel: [w767 w774] -> w765
        frame False {
          n214 = call "Fast_string_Replace.vi"("Replace match with:"="[", "Input String"=w768, "regular expression"="\\(") -> ("Output String"=w769:string)  [unwired: 1 in, 1 out]
          n215 = call "Fast_string_Replace.vi"("Replace match with:"="]", "Input String"=w769, "regular expression"="\\)") -> ("Output String"=w767:string)  [unwired: 1 in, 1 out]
        }
        frame True {
        }
      }
    }
  }
  "Channel Values Out" <- w4
